vi "PRIME Detector Send INIT.vi"(8 "error in (no error)":errorcluster, 11 "connection ID":refnum<k5>) -> (0 "error out":errorcluster, 3 "connection ID out":refnum<k5>)   [LabVIEW 2021, in "PRIME Detector.lvclass"]
uses:
  PRIME Detector.lvclass
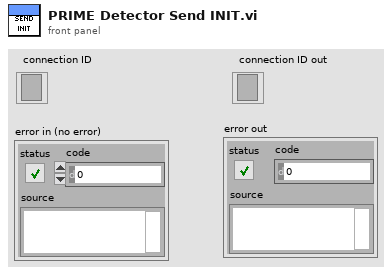
[diagram p1: front panel]
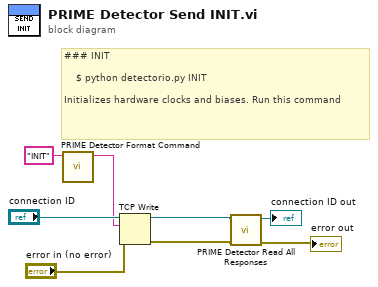
[diagram p0: block diagram]
diagram:
  # "### INIT\n\n    $ python detectorio.py INIT\n    \nInitializes hardware clocks and biases. Run this command"
  n1 = call "PRIME Detector Format Command.vi"("Command"="INIT") -> ("TCP String"=w6:string)  [unwired: 10 in]
  n2 = TCP Write(connection ID="connection ID", data in=w6, error in (no error)="error in (no error)") -> (connection ID out=w4:refnum<k5>, error out=w3:errorcluster)  [unwired: 1 in, 1 out]
  n3 = call "PRIME Detector Read All Responses.vi"("error in"=w3, "connection ID"=w4) -> ("error out"=→"error out":errorcluster, "connection ID out"=→"connection ID out":refnum<k5>)  [unwired: 6 in, 2 out]
